vi "step3 Solve.vi"(8 "error in (no error)":errorcluster, 11 "cube in":T1) -> (0 "error out":errorcluster, 1 "middle layer solved?":bool, 3 "cube out":T1)   [LabVIEW 2011]
doc: "Rotate cube as necessary so that the top middle piece matches the desired start colour.\n\nNo transformations are done in this VI, the operations are loaded on the the operation queue bus."
uses:
  Typedef/cube.ctl
  Typedef/face.ctl
  Typedef/operation.ctl
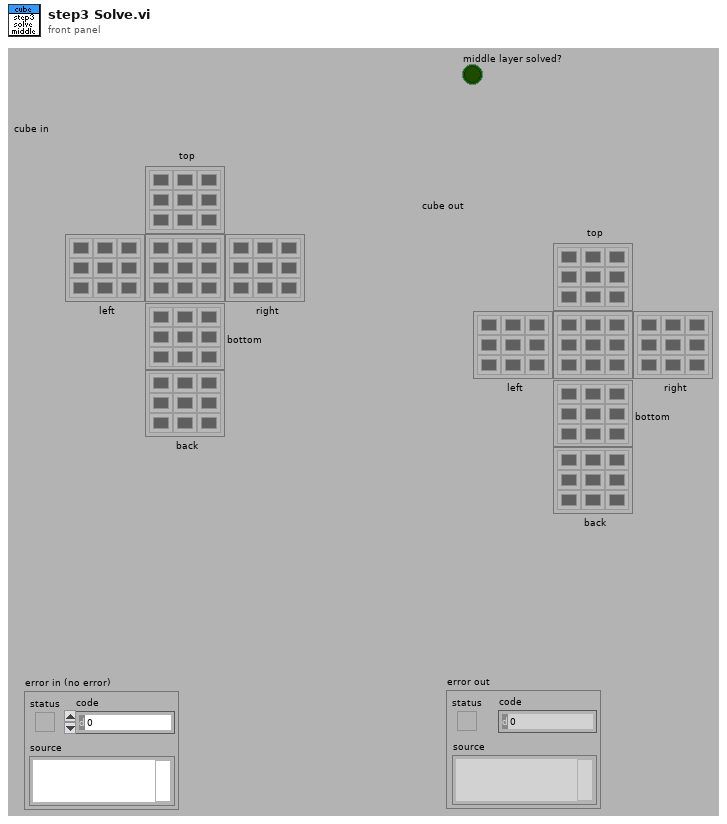
[diagram p1: front panel]
types:
  T1 = typedef "cube.ctl" = cluster{"top":T2, "left":T2, "right":T2, "bottom":T2, "back":T2, "front":T2}
  T2 = typedef "face.ctl" = u32[][]
  T3 = typedef "operation.ctl" = enum16{"nop", "T+", "T-", "F+", "F-", "L+", "L-", "R+", "R-", "B+", "B-", "<--", "-->", "^", "V"}
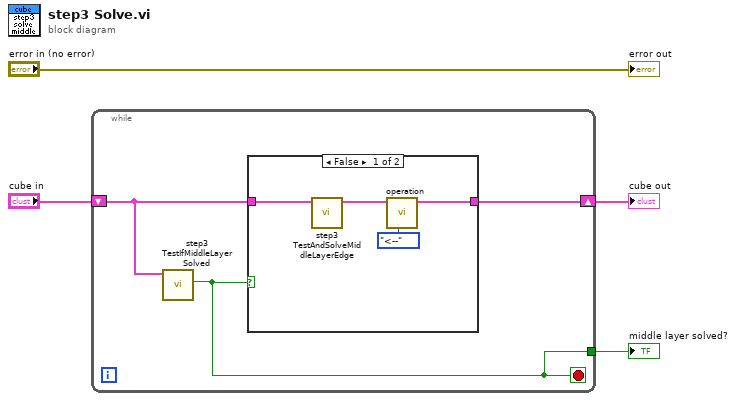
[diagram p0: block diagram]
diagram:
  n1 = while {
    shift-right: [w6] -> w2
    shift-left: "cube in" -> [w7]
    tunnel: [w5] -> w1
    stop <- w5 stop-if-true
    n2 = call "step3 TestIfMiddleLayerSolved.vi"("cube in"=w7) -> ("middle layer solved?"=w5:bool)  [unwired: 9 in, 1 out]
    n3 = case shown="False" w5 {
      tunnel: w7 -> [w10 w12]
      tunnel: [w8 w12] -> w6
      frame False {
        n4 = call "step3 TestAndSolveMiddleLayerEdge.vi"("cube in"=w10) -> ("cube out"=w9:T1)  [unwired: 10 in]
        n5 = call "operation.vi"("operation"=operation."<--", "cube in"=w9) -> ("cube out"=w8:T1)  [unwired: 8 in, 1 out]
      }
      frame True {
      }
    }
  }
  "middle layer solved?" <- w1
  "cube out" <- w2
  "error out" <- "error in (no error)"
